vi "Init blank volume table.vi"(8 "error in (no error)":errorcluster, 11 "Tomo in":refnum<class "Tomo.lvclass">) -> (0 "error out":errorcluster, 2 "blank volume table":dbl[][](array[numeric]), 3 "Tomo out":refnum<class "Tomo.lvclass">)   [LabVIEW 2012, in "Tomo.lvclass"]
uses:
  Tomo.lvclass
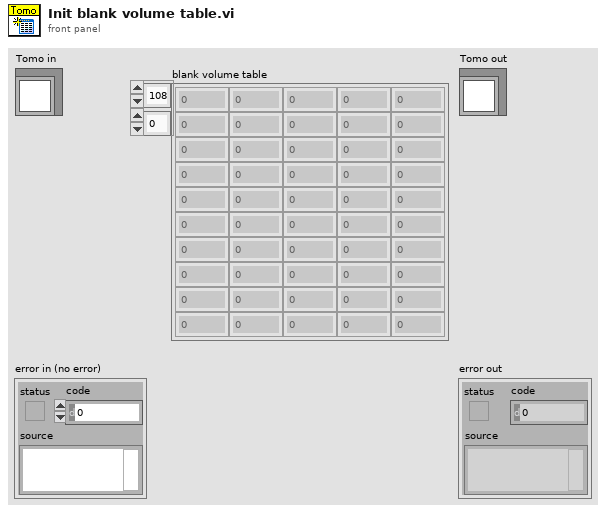
[diagram p1: front panel]
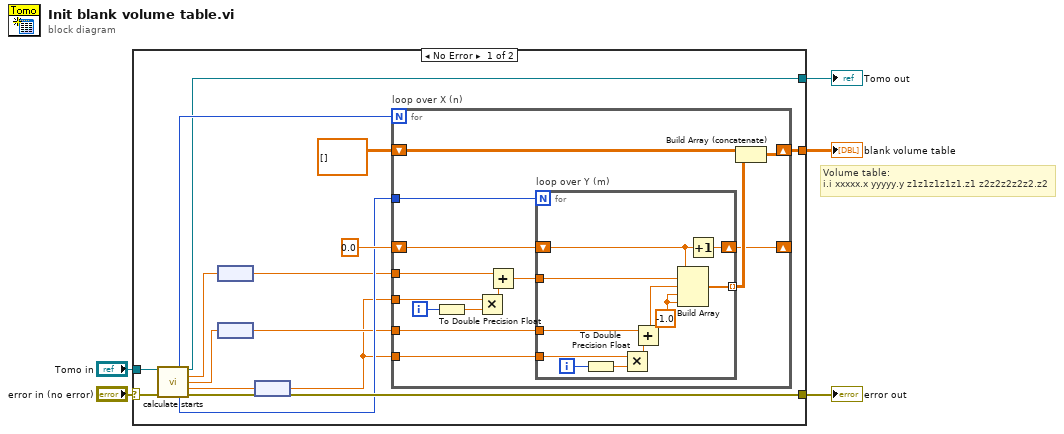
[diagram p0: block diagram]
diagram:
  # "Volume table: \ni.i xxxxx.x yyyyy.y z1z1z1z1z1.z1 z2z2z2z2z2.z2"
  n1 = case shown="No Error" "error in (no error)" {
    selector: "error in (no error)" -> [w17 w47]
    tunnel: [w16 w47] -> w4
    tunnel: [w7 w46] -> w2
    tunnel: "Tomo in" -> [w8 w46]
    tunnel: [w18 _] -> w1
    frame No Error {
      n2 = call-dynamic "calculate starts.vi"("Tomo in"=w8, "error in (no error)"=w17) -> ("x loop number"=w13:i32, "Tomo out"=w7:refnum<class "Tomo.lvclass">, "x_start"=w15:dbl[unit], "y_start"=w14:dbl[unit], "step size"=w9:dbl[unit], "y loop number"=w12:i32, "error out"=w16:errorcluster)  [unwired: 7 in]
      n3 = node(w15) -> (w11:dbl)
      n4 = node(w14) -> (w10:dbl)
      n5 = node(w9) -> (w6:dbl)
      n6 = for "loop over X (n)" {
        N: w13 -> [_]
        tunnel: w12 -> [w34]
        shift-right: [w21] -> _
        shift-left: 0.0 -> [w32]
        tunnel: w11 -> [w28]
        tunnel: w6 -> [w27]
        tunnel: w10 -> [w26]
        tunnel: w6 -> [w25]
        shift-right: [w24] -> w18
        shift-left: dbl[][] [] -> [w22]
        i -> [w33]
        n7 = To Double Precision Float(number=w33) -> (double precision float=w30:dbl)
        n8 = Multiply(x=w27, y=w30) -> (x*y=w31:dbl)
        n9 = Add(x=w28, y=w31) -> (x+y=w29:dbl)
        n10 = for "loop over Y (m)" {
          N: w34 -> [_]
          shift-right: [w44] -> w21
          shift-left: w32 -> [w36]
          tunnel: w29 -> [w43]
          tunnel: w26 -> [w42]
          tunnel: w25 -> [w41]
          tunnel: [w37] -> w23 mode=indexing
          i -> [w45]
          w35 = -1.0
          n11 = To Double Precision Float(number=w45) -> (double precision float=w40:dbl)
          n12 = Multiply(x=w41, y=w40) -> (x*y=w39:dbl)
          n13 = Add(x=w42, y=w39) -> (x+y=w38:dbl)
          n14 = Build Array(w36, w43, w38, w35, w35) -> (w37:dbl[])
          n15 = Increment(x=w36) -> (x+1=w44:dbl)
        }
        n16 = Build Array (concatenate)(w22, w23) -> (w24:dbl[][])
      }
    }
    frame Error {
    }
  }
  "error out" <- w4
  "Tomo out" <- w2
  "blank volume table" <- w1
